vi "Global 1.vi"() -> ()   [LabVIEW 2015]
panel:
  out "Intake Action":dbl
  in  "Climber State":dbl=10.0
  in  "Cancel Climb":bool
  in  "Auto-Climb":bool
  # "Global variables"
  # "Allowed values are:\n0 - idle\n10 - pickup to hold\n20 - hold to shooter\n30 - low shot\n40 - flush"
  # "The climber state reflects a state\nmachine. The path is in increasing\nnumerical order."
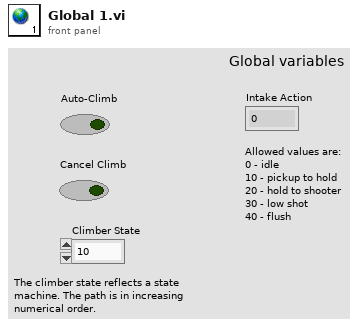
[diagram p1: front panel]
diagram:
